vi "Example-Lissajous-Figure.vi"() -> ()   [LabVIEW 2018]
panel:
  out "Scope -Lissajous":cluster{"voltages":dbl[], "voltages":dbl[]}(graph) caption="XY图"
  out "Scope Graph":cluster{"voltages":dbl[], "voltages":dbl[]}[](graph) caption="XY图"
  in  "trigcond":enum16{"Raising", "Falling", "Either"}(ring)
  in  "trigsrc":T1(ring)
  in  "trigtype":enum16{"edge", "pulse", "trasition"}(ring)
  in  "range 2":dbl=5.0
  in  "voltsLevel":dbl
  in  "timeout":i32
  in  "range":dbl=5.0
  in  "buffersize":i32=2048
  out "returns":i32[](array[numeric])
  in  "fre":i32=800000
  out "error out":errorcluster caption="错误输出"
  in  "error in (no error)":errorcluster caption="错误输入（无错误）"
  out "ftHandle out":u64=363562184
  in  "设备索引":i32
  # "0x0FFF"
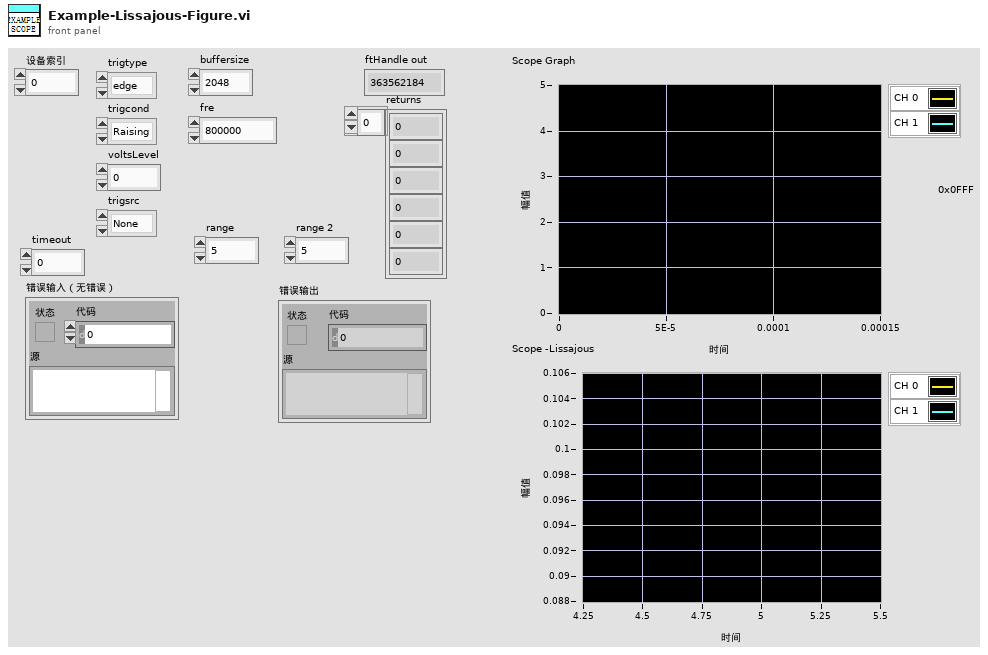
[diagram p1: front panel]
types:
  T1 = enum16{"None", "DetectorAnalogInCH1", "DetectorAnalogInCH2", "AnalogOut1", "AnalogOut2", "DetectorDigitalIn", "DigitalOut", "Manule", "External 1", "External 2", "DigitalIn"}
  T2 = enum16{"CLIFFStateReady", "CLIFFStateArmed", "CLIFFStateDone", "CLIFFStateRunning", "CLIFFStateConfig", "CLIFFStatePrefill", "CLIFFStateTriggered", "CLIFFStateWait"}
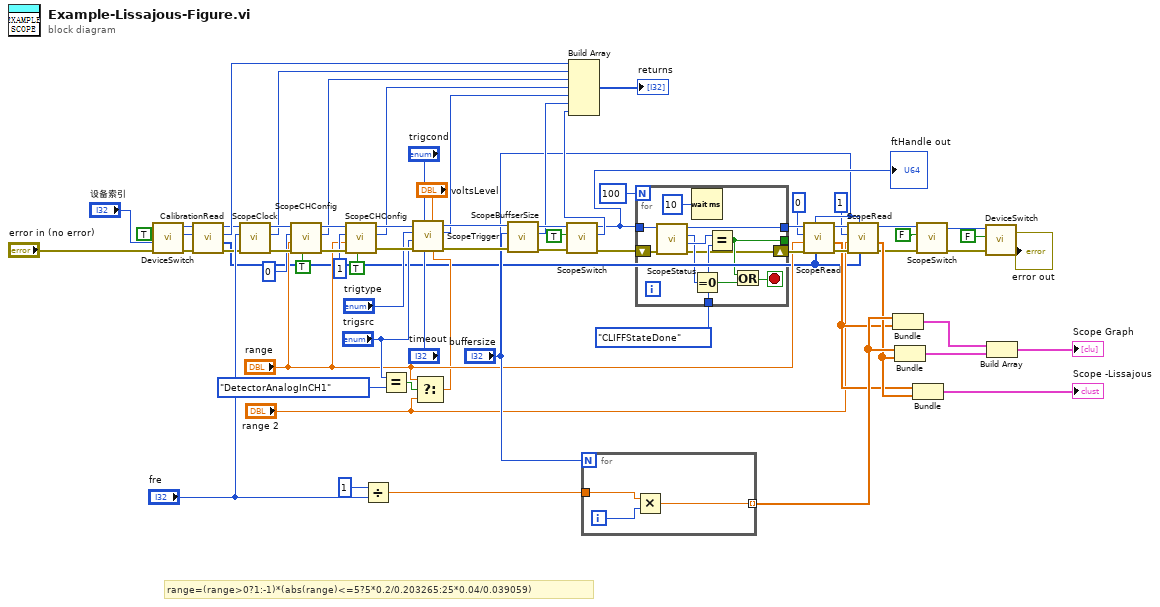
[diagram p0: block diagram]
diagram:
  # "range=(range>0?1:-1)*(abs(range)<=5?5*0.2/0.203265:25*0.04/0.039059)"
  n1 = call "DeviceSwitch.vi"("error in (no error)"="error in (no error)", "Device Index"="设备索引", "Open"=TRUE) -> ("error out"=w3:errorcluster, "function return"=w37:i32, "handle out"=w4:u64)  [unwired: 4 in, 2 out]
  n2 = call "CalibrationRead.vi"("handle"=w4, "error in (no error)"=w3) -> ("handle out"=w5:u64, "CalArray"=w1:u8[], "error out"=w2:errorcluster)  [unwired: 5 in, 1 out]
  n3 = call "ScopeClock.vi"("error in (no error)"=w2, "fre(Hz)"="fre", "handle"=w5) -> ("error out"=w49:errorcluster, "function return"=w36:i32, "handle out"=w58:u64)  [unwired: 6 in]
  n4 = call "ScopeCHConfig.vi"("enable"=TRUE, "error in (no error)"=w49, "range(V)"="range", "CH"=0 ("channel 3"), "handle"=w58) -> ("error out"=w48:errorcluster, "function return"=w35:i32, "handle out"=w59:u64)  [unwired: 4 in]
  n5 = call "ScopeCHConfig.vi"("enable"=TRUE, "error in (no error)"=w48, "range(V)"="range", "CH"=1 ("channel 2"), "handle"=w59) -> ("error out"=w56:errorcluster, "function return"=w34:i32, "handle out"=w57:u64)  [unwired: 4 in]
  n6 = Divide(x=1, y="fre") -> (x/y=w65:dbl)
  n7 = Equal?(x="trigsrc", y=T1."DetectorAnalogInCH1") -> (x = y?=w9:bool)
  n8 = Select(t="range", s=w9, f="range 2") -> (s? t:f=w6:dbl)
  n9 = call "ScopeTrigger.vi"("range"=w6, "voltsLevel"="voltsLevel", "timeout"="timeout", "trigcond"="trigcond", "error in (no error)"=w56, "trigsrc"="trigsrc", "trigtype"="trigtype", "handle"=w57) -> ("error out"=w55:errorcluster, "function return"=w33:i32, "handle out"=w54:u64)  [unwired: 1 in]
  n10 = call "ScopeBuffserSize.vi"("error in (no error)"=w55, "BufferSize"="buffersize", "handle"=w54) -> ("error out"=w47:errorcluster, "function return"=w32:i32, "handle out"=w53:u64)  [unwired: 6 in]
  n11 = call "ScopeSwitch.vi"("error in (no error)"=w47, "Run"=TRUE ("run"), "handle"=w53) -> ("error out"=w38:errorcluster, "function return"=w31:i32, "handle out"=w30:u64)  [unwired: 6 in]
  "ftHandle out" <- w30
  n12 = Build Array(w37, w36, w35, w34, w33, w32, w31) -> (→"returns":i32[])
  n13 = for {
    N: "buffersize" -> [_]
    tunnel: w65 -> [w71]
    tunnel: [w70] -> w61 mode=indexing
    i -> [w72]
    n14 = Multiply(x=w71, y=w72) -> (x*y=w70:dbl)
  }
  n15 = for {
    N: 100 -> [_]
    tunnel: w30 -> [w77]
    shift-right: [w73] -> w23
    shift-left: w38 -> [w78]
    tunnel: T2."CLIFFStateDone" ("ANIStatus") -> [w83]
    tunnel: [w76] -> w24
    tunnel: [w82] -> _
    stop <- w80 stop-if-true
    n16 = call "ScopeStatus.vi"("error in (no error)"=w78, "handle"=w77) -> ("error out"=w73:errorcluster, "ANIStatus"=w75:T2, "function return"=w74:i32, "handle out"=w76:u64)  [unwired: 6 in]
    n17 = Wait (ms)(milliseconds to wait=u32 10 ("等待时间（毫秒）")) -> ()  [unwired: 1 out]
    n18 = Equal To 0?(x=w74) -> (x = 0?=w79:bool)
    n19 = Equal?(x=w75, y=w83) -> (x = y?=w82:bool)
    n20 = Or(x=w82, y=w79) -> (x .or. y?=w80:bool)
  }
  n21 = call "ScopeRead.vi"("CalArray"=w1, "BufferSize"="buffersize", "error in (no error)"=w23, "Range"="range", "ch"=0, "handle"=w24) -> ("error out"=w26:errorcluster, "voltages"=w19:dbl[], "handle out"=w25:u64)  [unwired: 1 in, 2 out]
  n22 = call "ScopeRead.vi"("CalArray"=w1, "BufferSize"="buffersize", "error in (no error)"=w26, "Range"="range 2", "ch"=1, "handle"=w25) -> ("error out"=w12:errorcluster, "voltages"=w20:dbl[], "handle out"=w13:u64)  [unwired: 1 in, 2 out]
  n23 = Bundle(w61, "voltages"=w19) -> (w64:cluster{dbl[], "voltages":dbl[]})  [unwired: 1 in]
  n24 = Bundle(w61, "voltages"=w20) -> (w63:cluster{dbl[], "voltages":dbl[]})  [unwired: 1 in]
  n25 = Bundle("voltages"=w19, "voltages"=w20) -> (→"Scope -Lissajous":cluster{"voltages":dbl[], "voltages":dbl[]})  [unwired: 1 in]
  n26 = call "ScopeSwitch.vi"("error in (no error)"=w12, "Run"=FALSE, "handle"=w13) -> ("error out"=w15:errorcluster, "handle out"=w14:u64)  [unwired: 6 in, 1 out]
  n27 = call "DeviceSwitch.vi"("error in (no error)"=w15, "Open"=FALSE, "handle"=w14) -> ("error out"=→"error out":errorcluster)  [unwired: 4 in, 4 out]
  n28 = Build Array(w64, w63) -> (→"Scope Graph":cluster{dbl[], "voltages":dbl[]}[])
